vi "GOOP300_FindFilesToExchange.vi"(0 "OldClassName(Prefix or suffix for some VIs)":string="NotUsedIfNotWired", 1 "OldFolderPath":path, 2 "NewFolderPath":path, 3 "NewClassName(Prefix or suffix for some VIs)":string="NotUsedIfNotWired") -> (15 "OldFiles":path[](array[path]), 16 "NewFileArray":path[](array[path]))   [LabVIEW 2012]
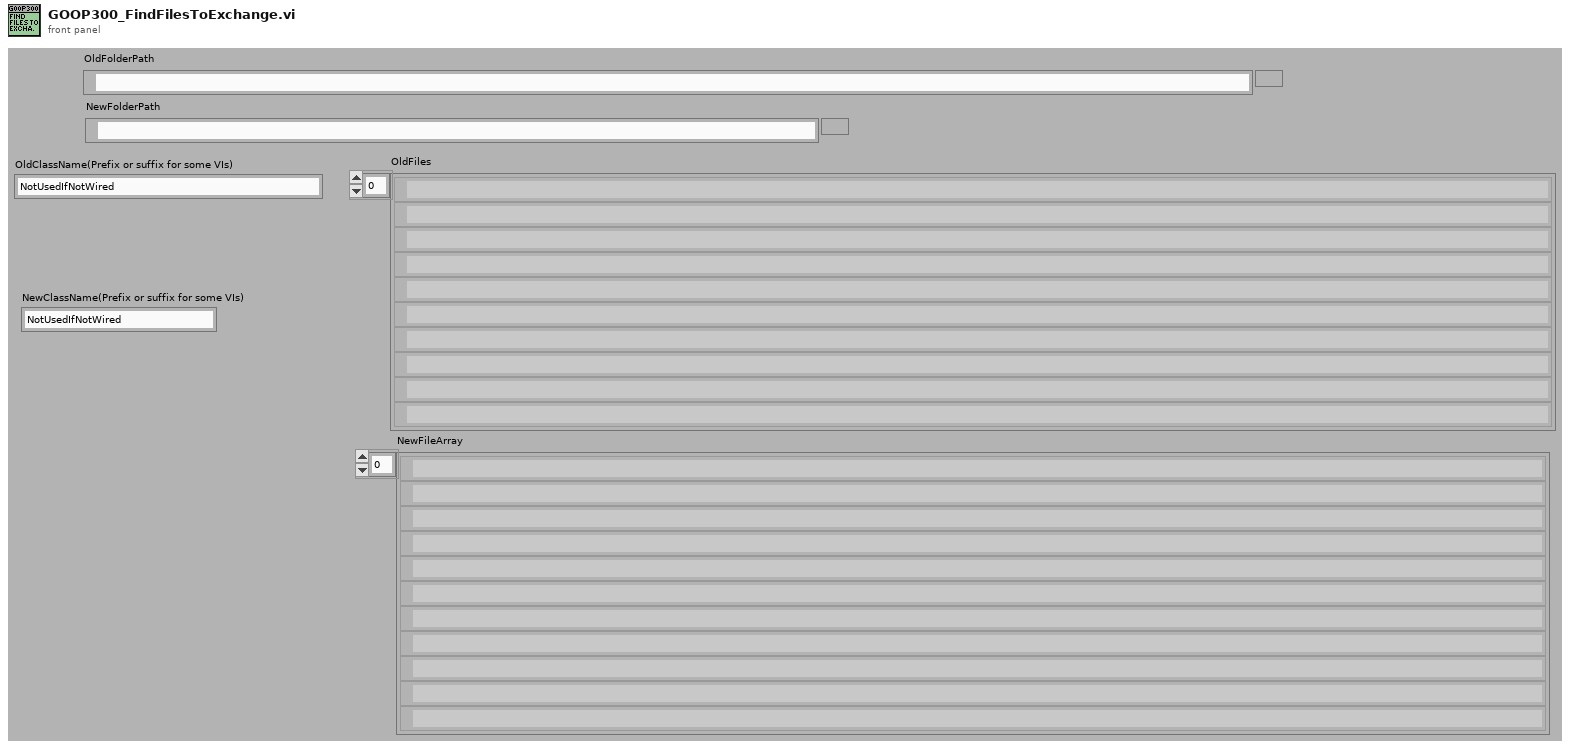
[diagram p1: front panel]
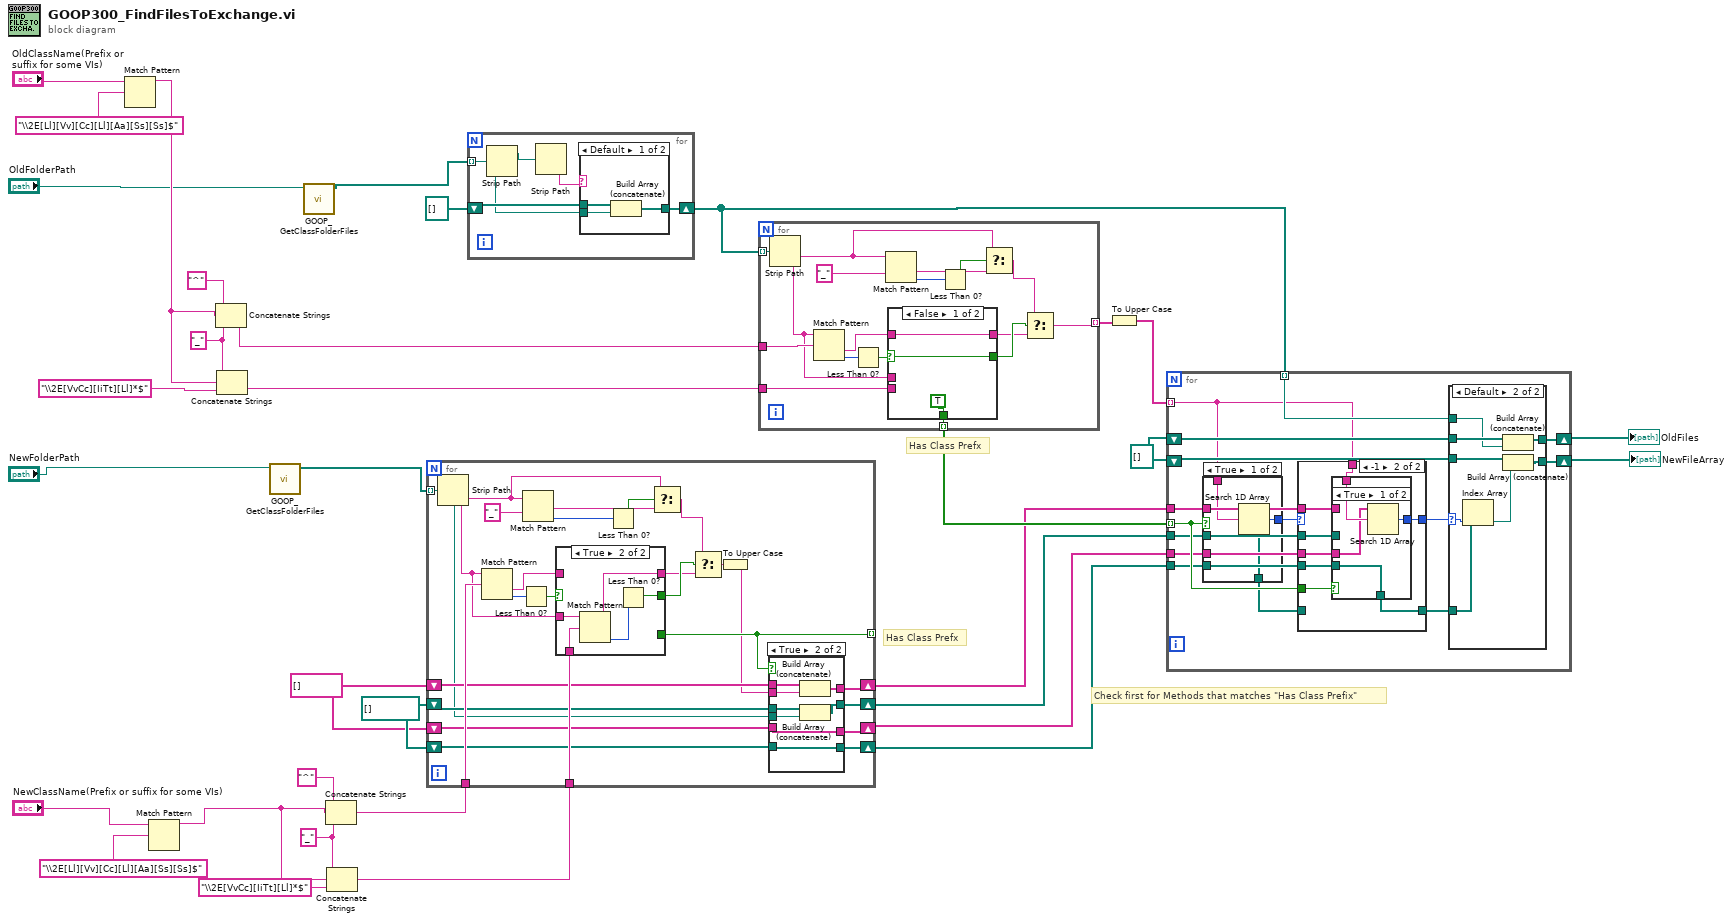
[diagram p0: block diagram]
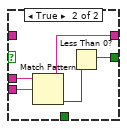
[diagram p2: hidden frame]
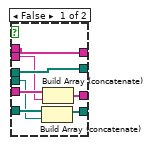
[diagram p3: hidden frame]
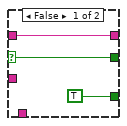
[diagram p4: hidden frame]
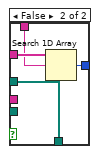
[diagram p6: hidden frame]
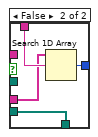
[diagram p7: hidden frame]
diagram:
  w12 = path[] []
  w11 = string[] []
  w17 = "_" ("regular expression")
  w29 = "_" ("regular expression")
  w32 = path[] []
  # "Check first for Methods that matches \"Has Class Prefix\""
  # "Has Class Prefx"
  # "Has Class Prefx"
  n1 = Match Pattern(string="OldClassName(Prefix or suffix for some VIs)", regular expression="\\2E[Ll][Vv][Cc][Ll][Aa][Ss][Ss]$") -> (before substring=w16:string)  [unwired: 1 in, 3 out]
  n2 = Match Pattern(string="NewClassName(Prefix or suffix for some VIs)", regular expression="\\2E[Ll][Vv][Cc][Ll][Aa][Ss][Ss]$") -> (before substring=w23:string)  [unwired: 1 in, 3 out]
  n3 = Concatenate Strings("^" ("string"), w16, w17) -> (w15:string)
  n4 = Concatenate Strings(w17, w16, "\\2E[VvCc][IiTt][Ll]*$" ("string")) -> (w14:string)
  n5 = call <resource>:"GOOP_GetClassFolderFiles.vi"("NewFolderPath"="NewFolderPath") -> ("Array"=w5:path[])  [unwired: 10 in]
  n6 = call <resource>:"GOOP_GetClassFolderFiles.vi"("NewFolderPath"="OldFolderPath") -> ("Array"=w1:path[])  [unwired: 10 in]
  n7 = Concatenate Strings("^" ("string"), w23, w29) -> (w30:string)
  n8 = Concatenate Strings(w29, w23, "\\2E[VvCc][IiTt][Ll]*$" ("string")) -> (w26:string)
  n9 = for {
    tunnel: w5 -> [w43] mode=indexing
    tunnel: w30 -> [w56]
    tunnel: w26 -> [w49]
    tunnel: [w41] -> _ mode=indexing
    shift-right: [w45] -> w7
    shift-left: w11 -> [w46]
    shift-right: [w42] -> w6
    shift-left: w12 -> [w44]
    shift-right: [w39] -> w4
    shift-left: w11 -> [w38]
    shift-right: [w40] -> w3
    shift-left: w12 -> [w37]
    n10 = Strip Path(path=w43) -> (name=w47:string)  [unwired: 1 out]
    n11 = Match Pattern(string=w47, regular expression=w56) -> (after substring=w51:string, offset past match=w55:i32)  [unwired: 1 in, 2 out]
    n12 = Less Than 0?(x=w55) -> (x < 0?=w53:bool)
    n13 = Match Pattern(string=w47, regular expression="_") -> (after substring=w48:string, offset past match=w59:i32)  [unwired: 1 in, 2 out]
    n14 = case shown="True" w53 {
      selector: w53 -> [w78 _]
      tunnel: [w78 w83] -> w52
      tunnel: w51 -> [w77 _]
      tunnel: [w77 w82] -> w50
      tunnel: w47 -> [_ w80]
      tunnel: w49 -> [_ w79]
      tunnel: [TRUE _] -> w41
      frame False {
      }
      frame True {
        n15 = Match Pattern(string=w80, regular expression=w79) -> (before substring=w82:string, offset past match=w81:i32)  [unwired: 1 in, 2 out]
        n16 = Less Than 0?(x=w81) -> (x < 0?=w83:bool)
      }
    }
    n17 = Less Than 0?(x=w59) -> (x < 0?=w58:bool)
    n18 = Select(t=w47, s=w58, f=w48) -> (s? t:f=w54:string)
    n19 = Select(t=w54, s=w52, f=w50) -> (s? t:f=w36:string)
    n20 = To Upper Case(1:w36) -> (0:w35:string)
    n21 = case shown="True" w41 {
      tunnel: w46 -> [w67 w75]
      tunnel: w35 -> [w61 w74]
      tunnel: [w67 w73] -> w45
      tunnel: w44 -> [w66 w72]
      tunnel: w43 -> [w60 w71]
      tunnel: [w66 w70] -> w42
      tunnel: [w65 w69] -> w39
      tunnel: [w64 w68] -> w40
      tunnel: w38 -> [w63 w69]
      tunnel: w37 -> [w62 w68]
      frame False {
        n22 = Build Array (concatenate)(w62, w60) -> (w64:path[])
        n23 = Build Array (concatenate)(w63, w61) -> (w65:string[])
      }
      frame True {
        n24 = Build Array (concatenate)(w75, w74) -> (w73:string[])
        n25 = Build Array (concatenate)(w72, w71) -> (w70:path[])
      }
    }
  }
  n26 = for {
    tunnel: w1 -> [w84] mode=indexing
    shift-right: [w85] -> w20
    shift-left: path[] [] -> [w86]
    n27 = Strip Path(path=w84) -> (stripped path=w88:path)  [unwired: 1 out]
    n28 = Strip Path(path=w88) -> (name=w87:string)  [unwired: 1 out]
    n29 = case shown="Default" w87 {
      tunnel: w86 -> [w91 w92]
      tunnel: [w90 w92] -> w85
      tunnel: w84 -> [w89 _]
      frame Default {
        n30 = Build Array (concatenate)(w91, w89) -> (w90:path[])
      }
      frame "Methods" {
      }
    }
  }
  n31 = for {
    tunnel: w20 -> [w108] mode=indexing
    tunnel: [w101] -> w10 mode=indexing
    tunnel: w15 -> [w96]
    tunnel: w14 -> [w95]
    tunnel: [w93] -> w8 mode=indexing
    n32 = Strip Path(path=w108) -> (name=w94:string)  [unwired: 1 out]
    n33 = Match Pattern(string=w94, regular expression=w96) -> (after substring=w98:string, offset past match=w103:i32)  [unwired: 1 in, 2 out]
    n34 = Less Than 0?(x=w103) -> (x < 0?=w100:bool)
    n35 = Match Pattern(string=w94, regular expression="_") -> (after substring=w106:string, offset past match=w107:i32)  [unwired: 1 in, 2 out]
    n36 = case shown="False" w100 {
      selector: w100 -> [w111 _]
      tunnel: [w111 w116] -> w99
      tunnel: w98 -> [w110 _]
      tunnel: [w110 w115] -> w97
      tunnel: w94 -> [_ w113]
      tunnel: w95 -> [_ w112]
      tunnel: [TRUE _] -> w93
      frame False {
      }
      frame True {
        n37 = Match Pattern(string=w113, regular expression=w112) -> (before substring=w115:string, offset past match=w114:i32)  [unwired: 1 in, 2 out]
        n38 = Less Than 0?(x=w114) -> (x < 0?=w116:bool)
      }
    }
    n39 = Less Than 0?(x=w107) -> (x < 0?=w105:bool)
    n40 = Select(t=w94, s=w105, f=w106) -> (s? t:f=w102:string)
    n41 = Select(t=w102, s=w99, f=w97) -> (s? t:f=w101:string)
  }
  n42 = To Upper Case(1:w10) -> (0:w9:string[])
  n43 = for {
    tunnel: w9 -> [w120] mode=indexing
    tunnel: w7 -> [w121]
    tunnel: w20 -> [w131] mode=indexing
    shift-right: [w129] -> w33
    shift-left: w32 -> [w130]
    shift-right: [w128] -> w34
    shift-left: w32 -> [w127]
    tunnel: w6 -> [w122]
    tunnel: w8 -> [w125] mode=indexing
    tunnel: w4 -> [w124]
    tunnel: w3 -> [w123]
    n44 = case shown="True" w125 {
      tunnel: w121 -> [w153 _]
      tunnel: [w152 w157] -> w126
      tunnel: w120 -> [w151 w156]
      tunnel: w122 -> [w150 _]
      tunnel: w124 -> [_ w155]
      tunnel: w123 -> [_ w154]
      tunnel: [w150 w154] -> w119
      frame True {
        n45 = Search 1D Array(1D array=w153, element=w151) -> (index of element=w152:i32)  [unwired: 1 in]
      }
      frame False {
        n46 = Search 1D Array(1D array=w155, element=w156) -> (index of element=w157:i32)  [unwired: 1 in]
      }
    }
    n47 = case shown="-1" w126 {
      selector: w126 -> [w132 _]
      tunnel: w125 -> [_ w141]
      tunnel: w124 -> [_ w140]
      tunnel: w123 -> [_ w139]
      tunnel: w122 -> [_ w138]
      tunnel: w121 -> [_ w137]
      tunnel: w120 -> [_ w136]
      tunnel: w119 -> [w133 _]
      tunnel: [w133 w134] -> w118
      tunnel: [w132 w135] -> w117
      frame 0, Default {
      }
      frame -1 {
        n48 = case shown="True" w141 {
          tunnel: w137 -> [_ w149]
          tunnel: [w145 w148] -> w135
          tunnel: w136 -> [w144 w147]
          tunnel: w138 -> [_ w146]
          tunnel: w140 -> [w143 _]
          tunnel: w139 -> [w142 _]
          tunnel: [w142 w146] -> w134
          frame True {
            n49 = Search 1D Array(1D array=w143, element=w144) -> (index of element=w145:i32)  [unwired: 1 in]
          }
          frame False {
            n50 = Search 1D Array(1D array=w149, element=w147) -> (index of element=w148:i32)  [unwired: 1 in]
          }
        }
      }
    }
    n51 = case shown="Default" w117 {
      selector: w117 -> [_ w162]
      tunnel: w131 -> [_ w166]
      tunnel: w130 -> [w158 w167]
      tunnel: [w158 w165] -> w129
      tunnel: [w159 w164] -> w128
      tunnel: w127 -> [w159 w163]
      tunnel: w118 -> [_ w160]
      frame -1 {
      }
      frame Default {
        n52 = Index Array(array=w160, index=w162) -> (element=w161:path)
        n53 = Build Array (concatenate)(w167, w166) -> (w165:path[])
        n54 = Build Array (concatenate)(w163, w161) -> (w164:path[])
      }
    }
  }
  "NewFileArray" <- w34
  "OldFiles" <- w33
